vi "TDMS to Patch Image.vi"(0 "Experiment Path":path, 11 "error in (no error)":errorcluster, 12 "Imaging Protocol":T2=enum."Functional Acquisition", 13 "Predominant ROI type":T1=enum."Rectangle", 14 "No of Patches in Experiment":i32) -> (4 "Current Trial Number":i32, 6 "Cancelled":bool, 10 "All Files in Dir":path[](array[path]), 15 "error out":errorcluster)   [LabVIEW 2013]
uses:
  Typedefs/Imaging Protocols enum.ctl
  Typedefs/ROI ID Enum.ctl
  Globals/gl_funct TIFF export globals.vi
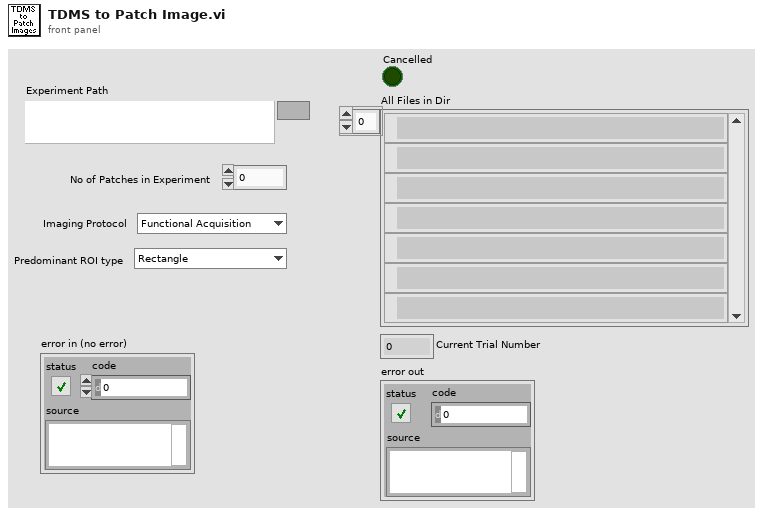
[diagram p1: front panel]
types:
  T1 = typedef "ROI ID Enum.ctl" = enum16{"Point", "MiniScan", "Comp. MiniScan", "Rectangle", "Comp. volume", "Arb. plane point"}
  T2 = typedef "Imaging Protocols enum.ctl" = enum16{"AOL Z-Stack", "Motor Z Stack", "Functional Acquisition", "Single Plane Acquisition", "Volume Acquisition", "Live Imaging", "Live Plane Imaging", "Live Volume Imaging"}
  T3 = typedef "Funct TIFF exporter ctrl refs.ctl" = cluster{"This VI":refnum<vi>, "Current Experiment":refnum<vi>, "Imaging protocol":refnum<vi>, "Predominant ROI type":refnum<vi>, "Patches in Experiment":refnum<vi>, "Folder Path":refnum<vi>, "Export":refnum<vi>, "Trial number":refnum<vi>, "Output TIFF type":refnum<vi>}
  T4 = typedef "Exported TIFF type.ctl" = enum16{"One multi-page TIFF file for each rectangle", "Individual TIFF files"}
  T5 = typedef "Fixed strings.ctl" = cluster{"ROI file name":string, "Normalised ROI file name":string, "Zplane Pockels values file name":string, "Functional data folder name":string, "Experiment Header file name":string, "Z-stack images folder name":string, "Groups setup rel. path":string, "Groups text file rel. path":string, "TDMS files folder name (F.img)":string, "TDMS files folder name (V.acq)":string, "TDMS files folder name (Pl.acq)":string, "Cycle rel times sequence file":string, "Dynamically called VIs folder name":string, "Time Series folder base name":string}
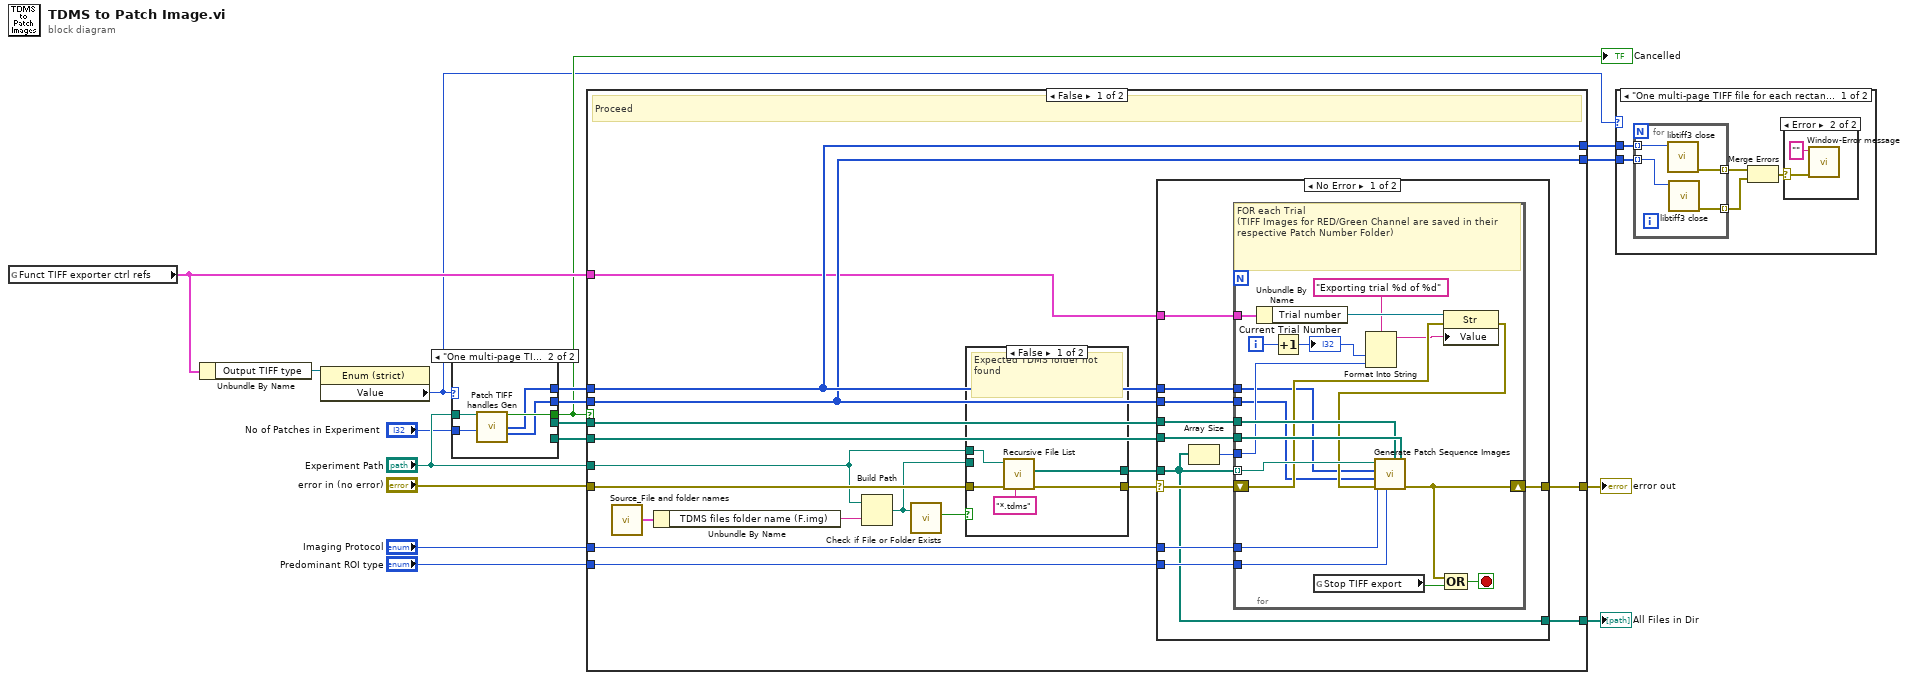
[diagram p0: block diagram]
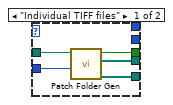
[diagram p4: hidden frame]
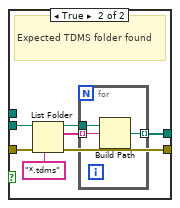
[diagram p5: hidden frame]
diagram:
  n1 = global read "gl_funct TIFF export globals.vi" "Funct TIFF exporter ctrl refs"() -> (w3:T3)
  n2 = Unbundle By Name(w3) -> ("Output TIFF type"=w4:refnum<vi>)
  n3 = property class="Enum (strict)"(reference=w4) -> ("Value"=w1:T4)  [unwired: 1 in, 2 out]
  n4 = case shown="\"One multi-page TIFF file for each rectangle\", Default" w1 {
    tunnel: [w22 _] -> w17
    tunnel: [w21 _] -> w16
    tunnel: [w20 w27] -> w2
    tunnel: "Experiment Path" -> [w19 w26]
    tunnel: "No of Patches in Experiment" -> [w18 w25]
    tunnel: [_ w24] -> w8
    tunnel: [_ w23] -> w7
    frame "Individual TIFF files" {
      n5 = call "Patch Folder Gen.vi"("No of Patches"=w18, "Experimental Folder"=w19) -> ("Green"=w21:path[], "Red"=w22:path[], "Cancelled"=w20:bool)  [unwired: 7 in]
    }
    frame "One multi-page TIFF file for each rectangle", Default {
      n6 = call "Patch TIFF handles Gen.vi"("Experimental Folder"=w26, "No of Patches"=w25) -> ("Cancelled"=w27:bool, "Red TIFF handles"=w24:i32[], "Green TIFF handles"=w23:i32[])  [unwired: 9 in, 2 out]
    }
  }
  "Cancelled" <- w2
  n7 = case shown="False" w2 {
    tunnel: w17 -> [w44 _]
    tunnel: w16 -> [w43 _]
    tunnel: "Imaging Protocol" -> [w42 _]
    tunnel: "Predominant ROI type" -> [w41 _]
    tunnel: [w40 w93] -> w12
    tunnel: "error in (no error)" -> [w38 w93]
    tunnel: [w39 _] -> w11
    tunnel: "Experiment Path" -> [w31 _]
    tunnel: w8 -> [w30 w92]
    tunnel: w7 -> [w29 w91]
    tunnel: [w30 w92] -> w6
    tunnel: [w29 w91] -> w5
    tunnel: w3 -> [w28 _]
    frame False {
      # "Proceed"
      n8 = call "Source_File and folder names.vi"() -> ("Fixed strings"=w35:T5)  [unwired: 1 in]
      n9 = Unbundle By Name(w35) -> ("TDMS files folder name (F.img)"=w34:string)
      n10 = Build Path(base path=w31, name or relative path=w34) -> (appended path=w32:path)
      n11 = call <vilib>:"Check if File or Folder Exists.vi"("path"=w32) -> ("file or folder exists?"=w33:bool)  [unwired: 8 in, 2 out]
      n12 = case shown="False" w33 {
        tunnel: w38 -> [w49 w56]
        tunnel: [w48 w55] -> w37
        tunnel: [w47 w50] -> w36
        tunnel: w32 -> [_ w54]
        tunnel: w31 -> [w45 _]
        frame False {
          # "Expected TDMS folder not found"
          n13 = call <vilib>:"Recursive File List.vi"("pattern"="*.tdms", "error in (no error)"=w49, "Folder Path"=w45) -> ("error out"=w48:errorcluster, "All Files in Dir"=w47:path[])  [unwired: 4 in, 3 out]
        }
        frame True {
          # "Expected TDMS folder found"
          n14 = List Folder(path=w54, pattern="*.tdms", error in=w56) -> (path out=w51:path, filenames=w52:string[], error out=w55:errorcluster)  [unwired: 1 in, 1 out]
          n15 = for {
            tunnel: w52 -> [w58] mode=indexing
            tunnel: w51 -> [w59]
            tunnel: [w57] -> w50 mode=indexing
            n16 = Build Path(base path=w59, name or relative path=w58) -> (appended path=w57:path)
          }
        }
      }
      n17 = case shown="No Error" w37 {
        selector: w37 -> [w65 w90]
        tunnel: w36 -> [w63 _]
        tunnel: w44 -> [w70 _]
        tunnel: w43 -> [w69 _]
        tunnel: w42 -> [w68 _]
        tunnel: w41 -> [w67 _]
        tunnel: [w66 w90] -> w40
        tunnel: [w63 _] -> w39
        tunnel: w28 -> [w64 _]
        tunnel: w30 -> [w61 _]
        tunnel: w29 -> [w60 _]
        frame No Error {
          n18 = Array Size(array=w63) -> (size(s)=w62:i32)
          n19 = for {
            tunnel: w63 -> [w89] mode=indexing
            tunnel: w70 -> [w87]
            tunnel: w69 -> [w88]
            tunnel: w68 -> [w86]
            tunnel: w67 -> [w85]
            shift-right: [w82] -> w66
            shift-left: w65 -> [w79]
            tunnel: w64 -> [w81]
            tunnel: w62 -> [w75]
            tunnel: w61 -> [w73]
            tunnel: w60 -> [w72]
            i -> [w71]
            stop <- w83 stop-if-true
            # "FOR each Trial\n(TIFF Images for RED/Green Channel are saved in their respective Patch Number Folder)"
            n20 = Unbundle By Name(w81) -> ("Trial number"=w80:refnum<vi>)
            n21 = Increment(x=w71) -> (x+1=w76:i32)
            "Current Trial Number" <- w76
            n22 = global read "gl_funct TIFF export globals.vi" "Stop TIFF export"() -> (w84:bool)
            n23 = Format Into String(format string="Exporting trial %d of %d", w76, w75) -> (resulting string=w74:string)  [unwired: 2 in, 1 out]
            n24 = property class="Str"(reference=w80, error in=w79, "Value"=w74) -> (error out=w78:errorcluster)  [unwired: 1 out]
            n25 = call "Generate Patch Sequence Images.vi"("Green"=w88, "Red"=w87, "Predominant ROI type"=w85, "Imaging Protocol"=w86, "error in (no error)"=w78, "Green TIFF handles"=w72, "Red TIFF handles"=w73, "TDMS file path & name"=w89) -> ("error out"=w82:errorcluster)  [unwired: 2 in, 1 out]
            n26 = Compound Arithmetic op=OR(w82, w84) -> (w83:bool)
          }
        }
        frame Error {
        }
      }
    }
    frame True {
      # "Error or cancelled"
    }
  }
  "error out" <- w12
  "All Files in Dir" <- w11
  n27 = case shown="\"One multi-page TIFF file for each rectangle\"" w1 {
    tunnel: w6 -> [w98 _]
    tunnel: w5 -> [w97 _]
    frame "One multi-page TIFF file for each rectangle" {
      n28 = for {
        tunnel: w98 -> [w104] mode=indexing
        tunnel: w97 -> [w103] mode=indexing
        tunnel: [w102] -> w95 mode=indexing
        tunnel: [w101] -> w96 mode=indexing
        n29 = call "libtiff3 close.vi"("Handle"=w104) -> ("error out"=w101:errorcluster)  [unwired: 9 in]
        n30 = call "libtiff3 close.vi"("Handle"=w103) -> ("error out"=w102:errorcluster)  [unwired: 9 in]
      }
      n31 = Merge Errors(w96, w95) -> (w94:errorcluster)
      n32 = case shown="Error" w94 {
        selector: w94 -> [_ w100]
        frame No Error {
        }
        frame Error {
          n33 = call "Window-Error message.vi"("error in (no error)"=w100, "Message"="") -> ()  [unwired: 9 in, 1 out]
        }
      }
    }
    frame "Individual TIFF files", Default {
    }
  }
